vi "Picolog Setup Channel.vi"(8 "Error In":errorcluster, 9 "Termocouple Type":T1=107 items=["B"=98, "E"=101, "J"=106, "K"=107, "N"=110, "R"=114, "S"=115, "T"=116, "Voltage"=120, "Internal"=0, "Off"=32], 10 "Channel":i16=6, 11 "Instrument Handle In":i16=1) -> (0 "Error Out":errorcluster, 3 "Instrument Handle Out":i16)   [LabVIEW 2017]
uses:
  Controls/Thermocouple.ctl
  usbtc08.dll
panel:
  out "Channel Out":i16
  out "Termocouple Type Out":i8
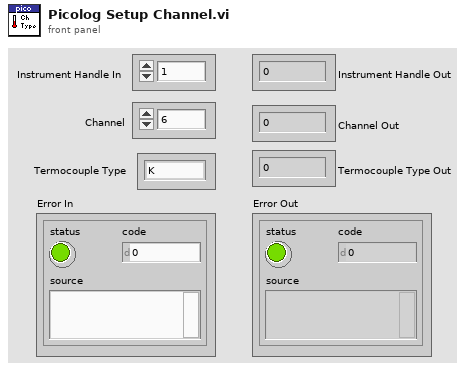
[diagram p1: front panel]
types:
  T1 = typedef "Thermocouple.ctl" = i8
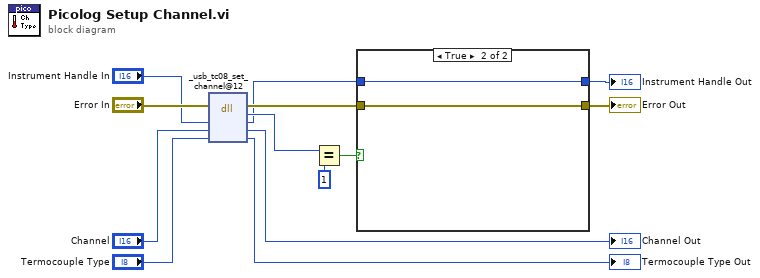
[diagram p0: block diagram]
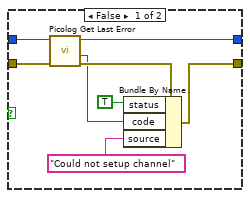
[diagram p2: hidden frame]
diagram:
  n1 = dll-call lib="usbtc08.dll" fn="_usb_tc08_set_channel@12"(error in="Error In", "handle"="Instrument Handle In", "channel"="Channel", "tc_type"="Termocouple Type") -> (error out=w5:errorcluster, "return type"=w7:i16, "handle"=w2:i16, "channel"=→"Channel Out":i16, "tc_type"=→"Termocouple Type Out":i8)  [unwired: 2 in, 1 out]
  n2 = Equal?(x=w7, y=i16 1 ("x")) -> (x = y?=w6:bool)
  n3 = case shown="True" w6 {
    tunnel: w5 -> [w19 w23]
    tunnel: [w21 w23] -> w4
    tunnel: w2 -> [w17 w22]
    tunnel: [w16 w22] -> w1
    frame False {
      n4 = call "Picolog Get Last Error.vi"("Error In"=w19, "Instrument Handle In"=w17) -> ("Error Out"=w18:errorcluster, "Error Code"=w14:i16, "Instrument Handle Out"=w16:i16)  [unwired: 7 in]
      n5 = Bundle By Name(cluster=w18, "status"=TRUE, "code"=w14, "source"="Could not setup channel") -> (w21:errorcluster)
    }
    frame True {
    }
  }
  "Error Out" <- w4
  "Instrument Handle Out" <- w1
